vi "20IOT4007 Harshraj Prasad.vi"() -> ()   [LabVIEW 2016]
doc: "The Simple PID Demo VI lets you see how a PID control system works without needing an external system to actually control. Run the VI. Notice with the default values you have a classic first order system reacting to a square wave. Try changing the System Type to 2nd ORDER and notice that the Process Variable does not track the Set Point very well. Try setting P=10, I=6, and D=5. Notice the difference as you tune the system. You can experiment withdifferent Set Point Types and tuning parameters to get a feel for tuning systems. View the help window description of each control for more information about its use."
panel:
  in  "Manual\nInput 2":dbl(slide) scale=-1.0..1.0 scale format="%.1f"
  in  "stop 2":bool
  out "chart 2":T1(graph)
  in  "Loop Delay\n(ms) 2":dbl(knob)=9.927881686189023 min=1.0 scale=0.0..50.0
  in  "tuning parameters 2":T2={"P"=1.2, "I"=25.0, "D"=0.0, "Upper Limit"=120.0, "Lower Limit"=-120.0} {"Lower Limit" format="%.3f"; "Upper Limit" format="%.3f"; "D" format="%.3f"; "I" format="%.3f"; "P" format="%.3f"}
  in  "menus 2":cluster{"Set Point Type":u16, "System Type":u16}={"Set Point Type"=3, "System Type"=0} {"System Type" items=["1st ORDER", "2nd ORDER"]; "Set Point Type" items=["SINE", "SINC", "ATAN", "SQUARE", "TRIANGLE", "SAWTOOTH", "RANDOM", "MANUAL"]}
  in  "menus":cluster{"Set Point Type":u16, "System Type":u16}={"Set Point Type"=3, "System Type"=0} {"System Type" items=["1st ORDER", "2nd ORDER"]; "Set Point Type" items=["SINE", "SINC", "ATAN", "SQUARE", "TRIANGLE", "SAWTOOTH", "RANDOM", "MANUAL"]}
  in  "Loop Delay\n(ms)":dbl(knob)=9.927881686189023 min=1.0 scale=0.0..50.0
  in  "Manual\nInput":dbl(slide) scale=-1.0..1.0 scale format="%.1f"
  out "chart":T1(graph)
  in  "stop":bool
  in  "tuning parameters":T2={"P"=1.2, "I"=25.0, "D"=0.0, "Upper Limit"=120.0, "Lower Limit"=-120.0} {"Lower Limit" format="%.3f"; "Upper Limit" format="%.3f"; "D" format="%.3f"; "I" format="%.3f"; "P" format="%.3f"}
  # "INPUT"
  # "OUTPUT"
  # "Set Point\n(what you\nwant)"
  # "Process\nVariable\n(what you\nare getting)"
  # "Tuning Parameters"
  # "Normalized\nPID Output"
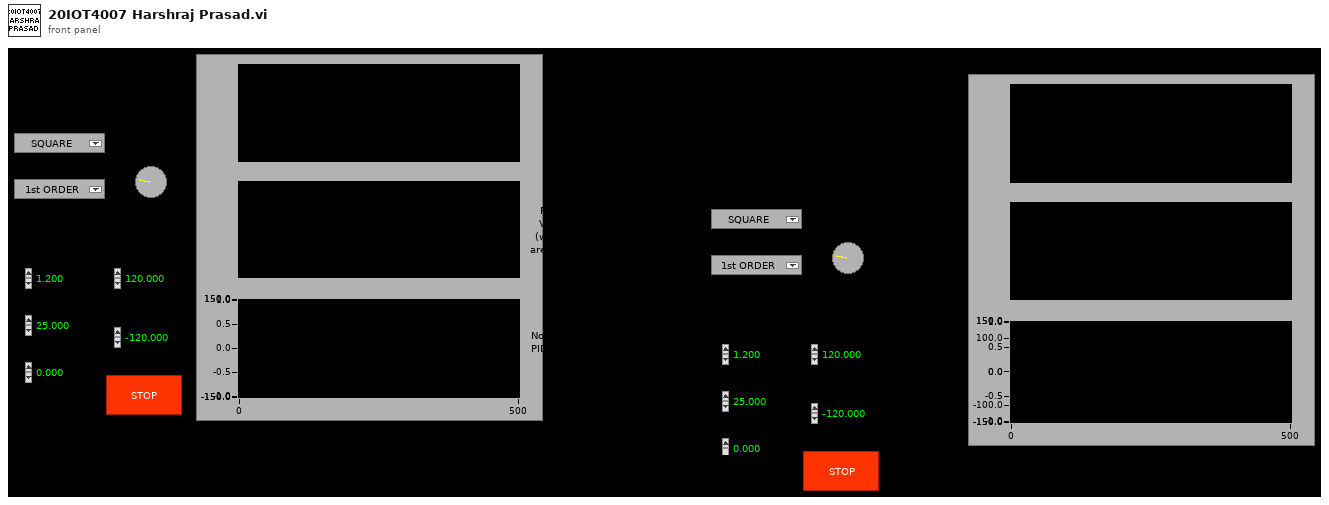
[diagram p1: front panel]
types:
  T1 = cluster{"setpoint":dbl, dbl, "normalized output value":dbl}
  T2 = cluster{"P":dbl, "I":dbl, "D":dbl, "Upper Limit":dbl, "Lower Limit":dbl}
  T3 = cluster{"set point":dbl, dbl, "normalized output value":dbl}
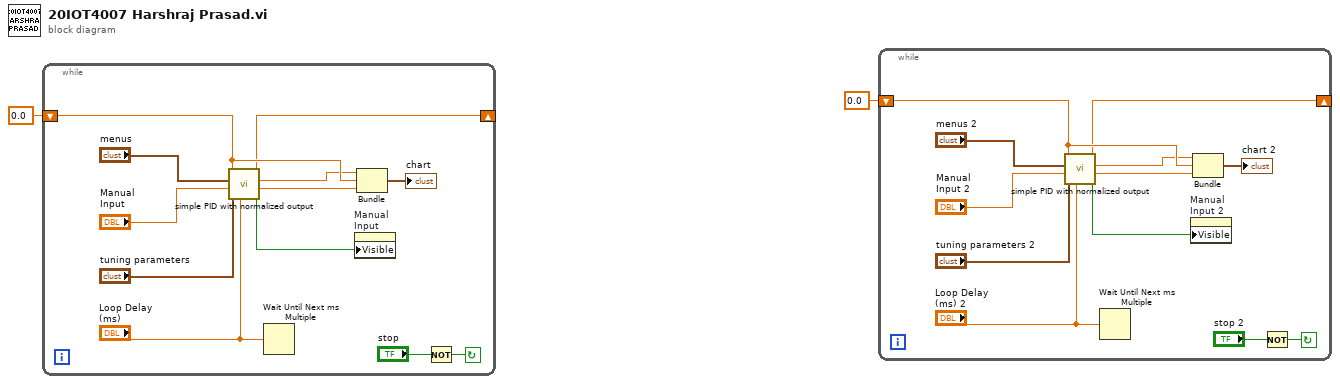
[diagram p0: block diagram]
diagram:
  n1 = while {
    shift-left: 0.0 -> [w10]
    shift-right: [w8] -> _
    stop <- w14 continue-if-true
    n2 = call "simple PID with normalized output.vi"("delta t (msec)"="Loop Delay\n(ms)", "tuning parameters"="tuning parameters", "manual input"="Manual\nInput", "menus"="menus", "process variable"=w10) -> ("show slider"=w6:bool, "normalized output value"=w7:dbl, "set point"=w9:dbl, "new process variable"=w8:dbl)  [unwired: 2 in, 1 out]
    n3 = Wait Until Next ms Multiple(millisecond multiple="Loop Delay\n(ms)") -> ()  [unwired: 1 out]
    n4 = property on="Manual\nInput" class="Slide (strict)"("Visible"=w6) -> ()  [unwired: 2 in, 2 out]
    n5 = Bundle("set point"=w9, w10, "normalized output value"=w7) -> (→"chart":T3)  [unwired: 1 in]
    n6 = Not(x="stop") -> (.not. x?=w14:bool)
  }
  n7 = while {
    shift-left: 0.0 -> [w22]
    shift-right: [w20] -> _
    stop <- w26 continue-if-true
    n8 = call "simple PID with normalized output.vi"("delta t (msec)"="Loop Delay\n(ms) 2", "tuning parameters"="tuning parameters 2", "manual input"="Manual\nInput 2", "menus"="menus 2", "process variable"=w22) -> ("show slider"=w18:bool, "normalized output value"=w19:dbl, "set point"=w21:dbl, "new process variable"=w20:dbl)  [unwired: 2 in, 1 out]
    n9 = Wait Until Next ms Multiple(millisecond multiple="Loop Delay\n(ms) 2") -> ()  [unwired: 1 out]
    n10 = property on="Manual\nInput 2" class="Slide (strict)"("Visible"=w18) -> ()  [unwired: 2 in, 2 out]
    n11 = Bundle("set point"=w21, w22, "normalized output value"=w19) -> (→"chart 2":T3)  [unwired: 1 in]
    n12 = Not(x="stop 2") -> (.not. x?=w26:bool)
  }
